vi "chart axis set name lv.vi"(8 "error in (no error)":errorcluster, 10 "name":string, 11 "axis":u32) -> (0 "error out":errorcluster)   [LabVIEW 2015, in "xlsxwriter.lvlib"]
doc: "void chart_axis_set_name_lv(lxw_chart_axis axis, const char *name);"
uses:
  xlsxwriter.lvlib
  xlsxwriter.dll
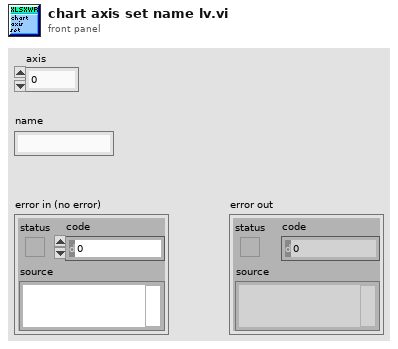
[diagram p1: front panel]
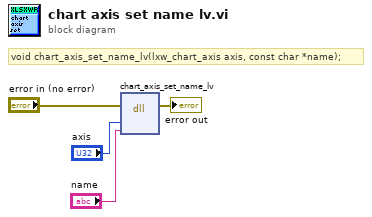
[diagram p0: block diagram]
diagram:
  # "void chart_axis_set_name_lv(lxw_chart_axis axis, const char *name);"
  n1 = dll-call lib="C:/Users/WDAGUtilityAccount/Desktop/lv_vis_added_cell/xlsxwriter.*" fn="chart_axis_set_name_lv"(error in="error in (no error)", "axis"="axis", "name"="name") -> (error out=→"error out":errorcluster)  [unwired: 5 in, 1 out]
